vi "Format Event Data.vi"(8 "error in":errorcluster, 9 "event array":T1[](array[typedef]) {"quality" items=["Good"=0, "Good_SubscriptionTransferred"=2949120, "Good_CompletesAsynchronously"=3014656, "Good_Overload"=3080192, "Good_Clamped"=3145728, "Good_LocalOverride"=9830400, "Good_EntryInserted"=10616832, "Good_EntryReplaced"=10682368, "Good_NoData"=10813440, "Good_MoreData"=10878976, "Good_CommunicationEvent"=10944512, "Good_ShutdownEvent"=11010048, "Good_CallAgain"=11075584, "Good_NonCriticalTimeout"=11141120, "Good_ResultsMayBeIncomplete"=12189696, "Good_DataIgnored"=14221312, "Uncertain"=1073741824, "Uncertain_ReferenceOutOfServer"=1080819712, "Uncertain_NoCommunicationLastUsableValue"=1083113472, "Uncertain_LastUsableValue"=1083179008, "Uncertain_SubstituteValue"=1083244544, "Uncertain_InitialValue"=1083310080, "Uncertain_SensorNotAccurate"=1083375616, "Uncertain_EngineeringUnitsExceeded"=1083441152, "Uncertain_SubNormal"=1083506688, "Uncertain_DataSubNormal"=1084489728, "Uncertain_ReferenceNotDeleted"=1086062592, "Uncertain_NotAllNodesAvailable"=1086324736, "Bad"=2147483648, "Bad_UnexpectedError"=2147549184, "Bad_InternalError"=2147614720, "Bad_OutOfMemory"=2147680256, "Bad_ResourceUnavailable"=2147745792, "Bad_CommunicationError"=2147811328, "Bad_EncodingError"=2147876864, "Bad_DecodingError"=2147942400, "Bad_EncodingLimitsExceeded"=2148007936, "Bad_UnknownResponse"=2148073472, "Bad_Timeout"=2148139008, "Bad_ServiceUnsupported"=2148204544, "Bad_Shutdown"=2148270080, "Bad_ServerNotConnected"=2148335616, "Bad_ServerHalted"=2148401152, "Bad_NothingToDo"=2148466688, "Bad_TooManyOperations"=2148532224, "Bad_DataTypeIdUnknown"=2148597760, "Bad_CertificateInvalid"=2148663296, "Bad_SecurityChecksFailed"=2148728832, "Bad_CertificateTimeInvalid"=2148794368, "Bad_CertificateIssuerTimeInvalid"=2148859904, "Bad_CertificateHostNameInvalid"=2148925440, "Bad_CertificateUriInvalid"=2148990976, "Bad_CertificateUseNotAllowed"=2149056512, "Bad_CertificateIssuerUseNotAllowed"=2149122048, "Bad_CertificateUntrusted"=2149187584, "Bad_CertificateRevocationUnknown"=2149253120, "Bad_CertificateIssuerRevocationUnknown"=2149318656, "Bad_CertificateRevoked"=2149384192, "Bad_CertificateIssuerRevoked"=2149449728, "Bad_UserAccessDenied"=2149515264, "Bad_IdentityTokenInvalid"=2149580800, "Bad_IdentityTokenRejected"=2149646336, "Bad_SecureChannelIdInvalid"=2149711872, "Bad_InvalidTimestamp"=2149777408, "Bad_NonceInvalid"=2149842944, "Bad_SessionIdInvalid"=2149908480, "Bad_SessionClosed"=2149974016, "Bad_SessionNotActivated"=2150039552, "Bad_SubscriptionIdInvalid"=2150105088, "Bad_RequestHeaderInvalid"=2150236160, "Bad_TimestampsToReturnInvalid"=2150301696, "Bad_RequestCancelledByClient"=2150367232, "Bad_NoCommunication"=2150694912, "Bad_WaitingForInitialData"=2150760448, "Bad_NodeIdInvalid"=2150825984, "Bad_NodeIdUnknown"=2150891520, "Bad_AttributeIdInvalid"=2150957056, "Bad_IndexRangeInvalid"=2151022592, "Bad_IndexRangeNoData"=2151088128, "Bad_DataEncodingInvalid"=2151153664, "Bad_DataEncodingUnsupported"=2151219200, "Bad_NotReadable"=2151284736, "Bad_NotWritable"=2151350272, "Bad_OutOfRange"=2151415808, "Bad_NotSupported"=2151481344, "Bad_NotFound"=2151546880, "Bad_ObjectDeleted"=2151612416, "Bad_NotImplemented"=2151677952, "Bad_MonitoringModeInvalid"=2151743488, "Bad_MonitoredItemIdInvalid"=2151809024, "Bad_MonitoredItemFilterInvalid"=2151874560, "Bad_MonitoredItemFilterUnsupported"=2151940096, "Bad_FilterNotAllowed"=2152005632, "Bad_StructureMissing"=2152071168, "Bad_EventFilterInvalid"=2152136704, "Bad_ContentFilterInvalid"=2152202240, "Bad_FilterOperandInvalid"=2152267776, "Bad_ContinuationPointInvalid"=2152333312, "Bad_NoContinuationPoints"=2152398848, "Bad_ReferenceTypeIdInvalid"=2152464384, "Bad_BrowseDirectionInvalid"=2152529920, "Bad_NodeNotInView"=2152595456, "Bad_ServerUriInvalid"=2152660992, "Bad_ServerNameMissing"=2152726528, "Bad_DiscoveryUrlMissing"=2152792064, "Bad_SempahoreFileMissing"=2152857600, "Bad_RequestTypeInvalid"=2152923136, "Bad_SecurityModeRejected"=2152988672, "Bad_SecurityPolicyRejected"=2153054208, "Bad_TooManySessions"=2153119744, "Bad_UserSignatureInvalid"=2153185280, "Bad_ApplicationSignatureInvalid"=2153250816, "Bad_NoValidCertificates"=2153316352, "Bad_RequestCancelledByRequest"=2153381888, "Bad_ParentNodeIdInvalid"=2153447424, "Bad_ReferenceNotAllowed"=2153512960, "Bad_NodeIdRejected"=2153578496, "Bad_NodeIdExists"=2153644032, "Bad_NodeClassInvalid"=2153709568, "Bad_BrowseNameInvalid"=2153775104, "Bad_BrowseNameDuplicated"=2153840640, "Bad_NodeAttributesInvalid"=2153906176, "Bad_TypeDefinitionInvalid"=2153971712, "Bad_SourceNodeIdInvalid"=2154037248, "Bad_TargetNodeIdInvalid"=2154102784, "Bad_DuplicateReferenceNotAllowed"=2154168320, "Bad_InvalidSelfReference"=2154233856, "Bad_ReferenceLocalOnly"=2154299392, "Bad_NoDeleteRights"=2154364928, "Bad_ServerIndexInvalid"=2154430464, "Bad_ViewIdUnknown"=2154496000, "Bad_TooManyMatches"=2154627072, "Bad_QueryTooComplex"=2154692608, "Bad_NoMatch"=2154758144, "Bad_MaxAgeInvalid"=2154823680, "Bad_HistoryOperationInvalid"=2154889216, "Bad_HistoryOperationUnsupported"=2154954752, "Bad_WriteNotSupported"=2155020288, "Bad_TypeMismatch"=2155085824, "Bad_MethodInvalid"=2155151360, "Bad_ArgumentsMissing"=2155216896, "Bad_TooManySubscriptions"=2155282432, "Bad_TooManyPublishRequests"=2155347968, "Bad_NoSubscription"=2155413504, "Bad_SequenceNumberUnknown"=2155479040, "Bad_MessageNotAvailable"=2155544576, "Bad_InsufficientClientProfile"=2155610112, "Bad_TcpServerTooBusy"=2155675648, "Bad_TcpMessageTypeInvalid"=2155741184, "Bad_TcpSecureChannelUnknown"=2155806720, "Bad_TcpMessageTooLarge"=2155872256, "Bad_TcpNotEnoughResources"=2155937792, "Bad_TcpInternalError"=2156003328, "Bad_TcpEndpointUrlInvalid"=2156068864, "Bad_RequestInterrupted"=2156134400, "Bad_RequestTimeout"=2156199936, "Bad_SecureChannelClosed"=2156265472, "Bad_SecureChannelTokenUnknown"=2156331008, "Bad_SequenceNumberInvalid"=2156396544, "Bad_ConfigurationError"=2156462080, "Bad_NotConnected"=2156527616, "Bad_DeviceFailure"=2156593152, "Bad_SensorFailure"=2156658688, "Bad_OutOfService"=2156724224, "Bad_DeadbandFilterInvalid"=2156789760, "Bad_RefreshInProgress"=2157379584, "Bad_ConditionAlreadyDisabled"=2157445120, "Bad_ConditionDisabled"=2157510656, "Bad_EventIdUnknown"=2157576192, "Bad_NoData"=2157641728, "Bad_DataLost"=2157772800, "Bad_DataUnavailable"=2157838336, "Bad_EntryExists"=2157903872, "Bad_NoEntryExists"=2157969408, "Bad_TimestampNotSupported"=2158034944, "Bad_InvalidArgument"=2158690304, "Bad_ConnectionRejected"=2158755840, "Bad_Disconnect"=2158821376, "Bad_ConnectionClosed"=2158886912, "Bad_InvalidState"=2158952448, "Bad_EndOfStream"=2159017984, "Bad_NoDataAvailable"=2159083520, "Bad_WaitingForResponse"=2159149056, "Bad_OperationAbandoned"=2159214592, "Bad_ExpectedStreamToBlock"=2159280128, "Bad_WouldBlock"=2159345664, "Bad_SyntaxError"=2159411200, "Bad_MaxConnectionsReached"=2159476736, "Bad_RequestTooLarge"=2159542272, "Bad_ResponseTooLarge"=2159607808, "Bad_EventNotAcknowledgeable"=2159738880, "Bad_InvalidTimestampArgument"=2159869952, "Bad_ProtocolVersionUnsupported"=2159935488, "Bad_StateNotActive"=2160001024, "Bad_FilterOperatorInvalid"=2160132096, "Bad_FilterOperatorUnsupported"=2160197632, "Bad_FilterOperandCountMismatch"=2160263168, "Bad_FilterElementInvalid"=2160328704, "Bad_FilterLiteralInvalid"=2160394240, "Bad_IdentityChangeNotSupported"=2160459776, "Bad_NotTypeDefinition"=2160590848, "Bad_ViewTimestampInvalid"=2160656384, "Bad_ViewParameterMismatch"=2160721920, "Bad_ViewVersionInvalid"=2160787456, "Bad_ConditionAlreadyEnabled"=2160852992, "Bad_DialogNotActive"=2160918528, "Bad_DialogResponseInvalid"=2160984064, "Bad_ConditionBranchAlreadyAcked"=2161049600, "Bad_ConditionBranchAlreadyConfirmed"=2161115136, "Bad_ConditionAlreadyShelved"=2161180672, "Bad_ConditionNotShelved"=2161246208, "Bad_ShelvingTimeOutOfRange"=2161311744, "Bad_AggregateListMismatch"=2161377280, "Bad_AggregateNotSupported"=2161442816, "Bad_AggregateInvalidInputs"=2161508352, "Bad_BoundNotFound"=2161573888, "Bad_BoundNotSupported"=2161639424, "Bad_AggregateConfigurationRejected"=2161770496, "Bad_TooManyMonitoredItems"=2161836032]}, 10 "type":enum16{"Insert", "Replace", "Append"}(ring), 11 "Multicolumn Listbox":refnum<vi>) -> (0 "error out":errorcluster, 1 "Alarm Summary Data":string[][](array[string]), 2 "Alarm Summary Headers":string[](array[string]), 3 "dup Multicolumn Listbox":refnum<vi>)   [LabVIEW 2019]
uses:
  Event Description Item.ctl
  <vilib>/OPCUA/controls/Event Fields.ctl
  <vilib>/OPCUA/controls/NodeId.ctl
  <vilib>/OPCUA/controls/Condition Type.ctl
  <vilib>/OPCUA/controls/OPC UA StatusCode.ctl
panel:
  in  "alarm display format":T5[](array[typedef])=[enum."acked state", enum."confrimed state", enum."time", enum."severity", enum."active", enum."source node ID", enum."condition node ID", enum."condition type", enum."comment", enum."event ID"]
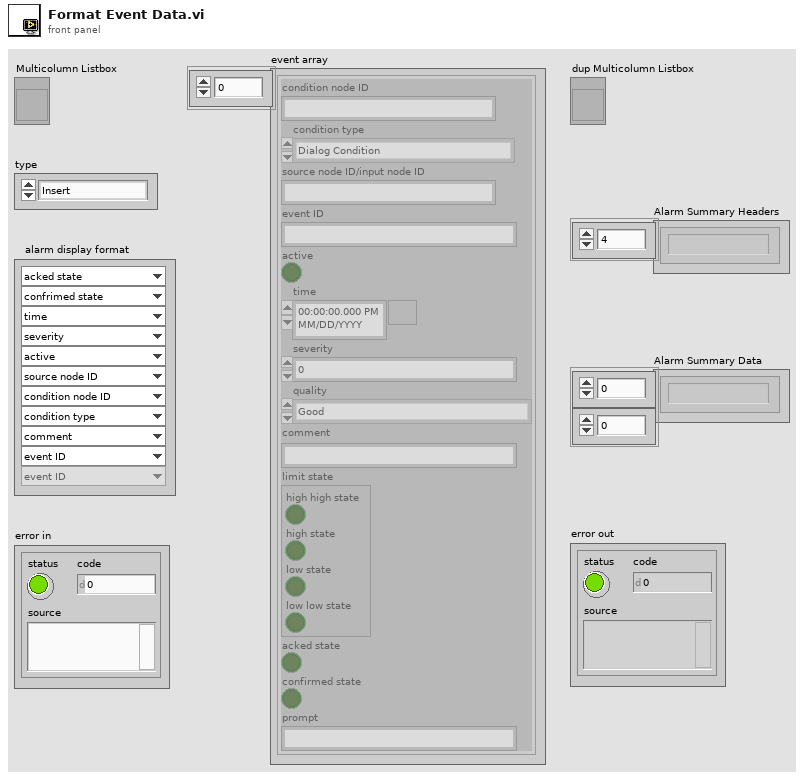
[diagram p1: front panel]
types:
  T1 = typedef "Event Fields.ctl" = cluster{"condition node ID":T2, "condition type":T3, "source node ID/input node ID":T2, "event ID":string, "active":bool, "time":timestamp, "severity":u16, "quality":T4, "comment":string, "limit state":cluster{"high high state":bool, "high state":bool, "low state":bool, "low low state":bool}, "acked state":bool, "confirmed state":bool, "prompt":string}
  T2 = typedef "NodeId.ctl" = string
  T3 = typedef "Condition Type.ctl" = enum16{"Dialog Condition", "Off-Normal Alarm", "Exclusive Level Alarm", "Exclusive Deviation Alarm", "Exclusive Rate of Change Alarm", "Nonexclusive Level Alarm", "Nonexclusive Deviation Alarm", "Nonexclusive Rate of Change Alarm", "Refresh Start Event", "Refresh End Event"}
  T4 = typedef "OPC UA StatusCode.ctl" = u32
  T5 = typedef "Event Description Item.ctl" = enum16{"event ID", "active", "condition type", "condition node ID", "source node ID", "time", "severity", "quality", "comment", "high high state", "high state", "low state", "low low state", "acked state", "confrimed state", "prompt"}
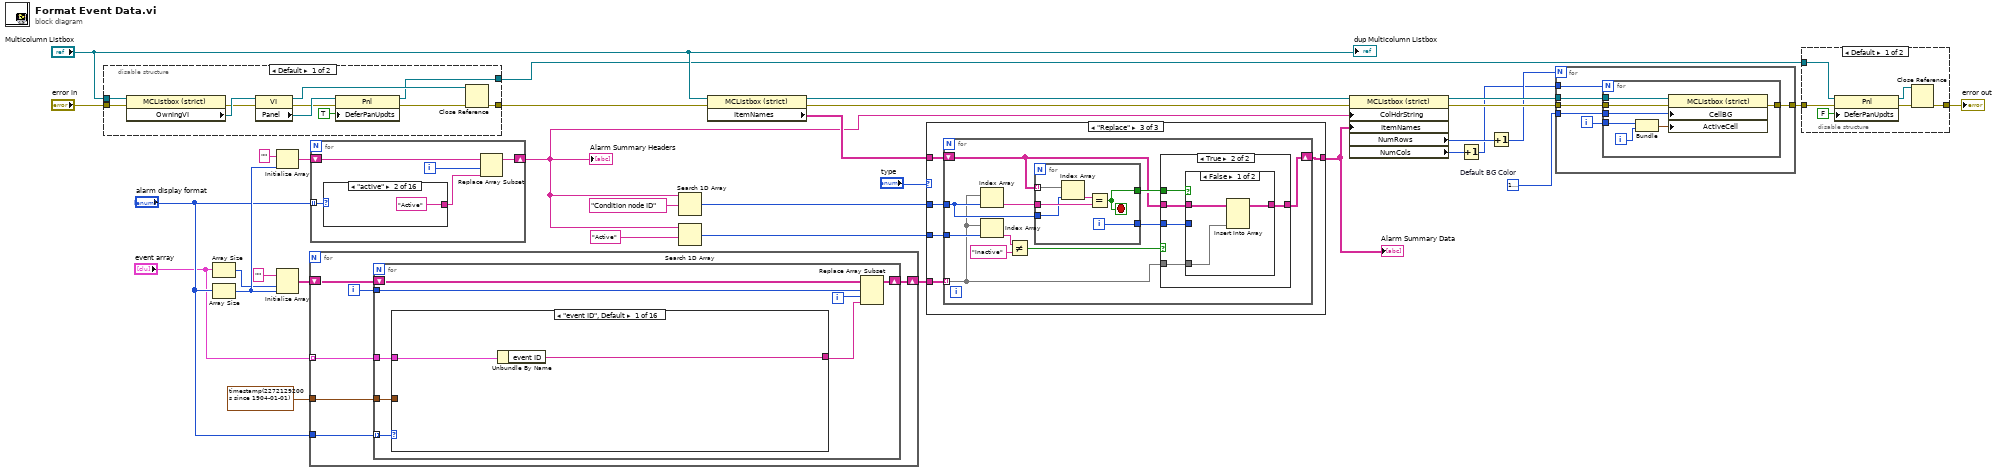
[diagram p0: block diagram]
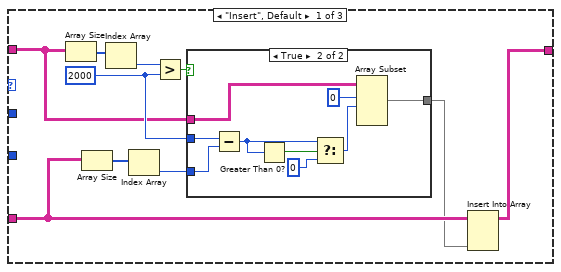
[diagram p4: hidden frame]
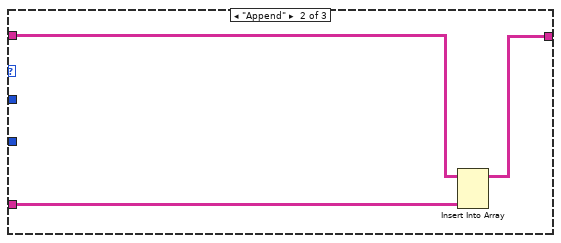
[diagram p6: hidden frame]
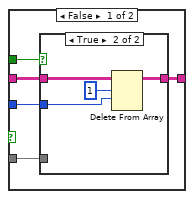
[diagram p7: hidden frame]
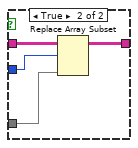
[diagram p9: hidden frame]
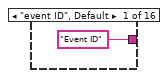
[diagram p10: hidden frame]
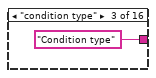
[diagram p11: hidden frame]
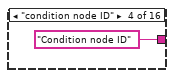
[diagram p12: hidden frame]
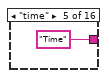
[diagram p13: hidden frame]
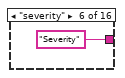
[diagram p14: hidden frame]
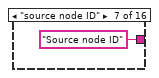
[diagram p15: hidden frame]
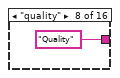
[diagram p16: hidden frame]
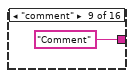
[diagram p17: hidden frame]
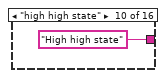
[diagram p18: hidden frame]
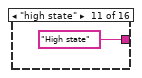
[diagram p19: hidden frame]
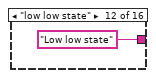
[diagram p20: hidden frame]
diagram:
  w19 = u32 16777226  # Default BG Color
  n1 = disable-structure shown="Default" {
    disable-tunnel: "error in" -> [w37 w45]
    disable-tunnel: "Multicolumn Listbox" -> [w36 _]
    disable-tunnel: [w35 w45] -> w5
    disable-tunnel: [w34 _] -> w2
    frame condition #0 (active) {
      n2 = property class="MCListbox (strict)"(reference=w36, error in=w37) -> (error out=w43:errorcluster, "OwningVI"=w44:refnum<vi>)  [unwired: 1 out]
      n3 = property class="VI"(reference=w44, error in=w43) -> (reference out=w39:refnum<vi>, error out=w41:errorcluster, "Panel"=w42:refnum<vi>)
      n4 = property class="Pnl"(reference=w42, error in=w41, "DeferPanUpdts"=TRUE ("Defer Panel Updates")) -> (reference out=w34:refnum<vi>, error out=w38:errorcluster)
      n5 = Close Reference(reference=w39, error in (no error)=w38) -> (error out=w35:errorcluster)
    }
    frame condition #1 {
    }
  }
  n6 = Array Size(array="event array") -> (size(s)=w28:i32)
  n7 = Array Size(array="alarm display format") -> (size(s)=w32:i32)
  n8 = Initialize Array("" ("element"), w32) -> (w33:string[])
  n9 = Initialize Array("" ("alarm URL"), w28, w32) -> (w30:string[][])
  n10 = for {
    tunnel: "event array" -> [w46] mode=indexing
    tunnel: "alarm display format" -> [w51]
    shift-right: [w49] -> w13
    shift-left: w30 -> [w50]
    tunnel: timestamp(2272129200 s since 1904-01-01) ("ack time") -> [w47]
    i -> [w48]
    n11 = for {
      tunnel: w51 -> [w59] mode=indexing
      tunnel: w46 -> [w52]
      tunnel: w48 -> [w56]
      shift-right: [w57] -> w49
      shift-left: w50 -> [w58]
      tunnel: w47 -> [w53]
      i -> [w55]
      n12 = case shown="\"event ID\", Default" w59 {
        tunnel: w52 -> [w61 w63 w64 w83 w88 w95 w108 w111 w113 w118 w123 w128 w133 w138 w143 w145]
        tunnel: [w60 w62 w65 w82 w87 w94 w106 w109 w112 w114 w119 w124 w129 w134 w139 w144] -> w54
        tunnel: w53 -> [_ _ _ _ w85 _ _ _ _ _ _ _ _ _ _ _]
        frame "event ID", Default {
          n13 = Unbundle By Name(w61) -> ("event ID"=w60:string)
        }
        frame "source node ID" {
          n14 = Unbundle By Name(w63) -> ("source node ID/input node ID"=w62:T2)
        }
        frame "active" {
          n15 = Unbundle By Name(w64) -> ("active"=w66:bool)
          n16 = case shown="True" w66 {
            tunnel: ["Inactive" ("f") w68] -> w65
            tunnel: w64 -> [_ w77]
            frame False {
            }
            frame True {
              n17 = Unbundle By Name(w77) -> ("limit state.high high state"=w76:bool, "limit state.high state"=w75:bool, "limit state.low state"=w74:bool, "limit state.low low state"=w73:bool)
              n18 = Build Array(w76, w75, w74, w73) -> (w72:bool[])
              n19 = Boolean Array To Number(Boolean array=w72) -> (number=w71:u32)
              n20 = case shown="8, 12" w71 {
                tunnel: ["HighHigh" ("f") "High" ("f") "Low" ("f") "LowLow" ("f")] -> w69
                frame 1, 3, Default {
                }
                frame 2 {
                }
                frame 4 {
                }
                frame 8, 12 {
                }
              }
              n21 = Concatenate Strings("Active | " ("f"), w69) -> (w68:string)
            }
          }
        }
        frame "condition node ID" {
          n22 = Unbundle By Name(w83) -> ("condition node ID"=w82:T2)
        }
        frame "time" {
          n23 = Unbundle By Name(w88) -> ("time"=w84:timestamp)
          n24 = Less?(x=w84, y=w85) -> (x < y?=w86:bool)
          n25 = case shown="True" w86 {
            tunnel: w84 -> [w91 _]
            tunnel: [w89 "" ("date/time string")] -> w87
            frame False {
              n26 = Format Date/Time String(time format string (%c)="%m/%d/%Y %H:%M:%S", seconds (now)=w91) -> (date/time string=w89:string)  [unwired: 1 in]
            }
            frame True {
            }
          }
        }
        frame "condition type" {
          n27 = Unbundle By Name(w95) -> ("condition type"=w93:T3)
          n28 = case shown="\"Exclusive Level Alarm\"" w93 {
            tunnel: ["Dialog Condition" ("alarm URL") "Off Normal Alarm" ("alarm URL") "Exclusive Level Alarm" ("alarm URL") "Exclusive Deviation Alarm" ("alarm URL") "Exclusive Rate of Change Alarm" ("alarm URL") "Nonexclusive Level Alarm" ("alarm URL") "Nonexclusive Deviation Alarm" ("alarm URL") "Nonexclusive Rate of Change Alarm" ("alarm URL") "Refresh Start Event" ("alarm URL") "Refresh End Event" ("alarm URL")] -> w94
            frame "Dialog Condition", Default {
            }
            frame "Off-Normal Alarm" {
            }
            frame "Exclusive Level Alarm" {
            }
            frame "Exclusive Deviation Alarm" {
            }
            frame "Exclusive Rate of Change Alarm" {
            }
            frame "Nonexclusive Level Alarm" {
            }
            frame "Nonexclusive Deviation Alarm" {
            }
            frame "Nonexclusive Rate of Change Alarm" {
            }
            frame "Refresh Start Event" {
            }
            frame "Refresh End Event" {
            }
          }
        }
        frame "severity" {
          n29 = Unbundle By Name(w108) -> ("severity"=w107:u16)
          n30 = Number To Decimal String(number=w107) -> (decimal integer string=w106:string)  [unwired: 1 in]
        }
        frame "quality" {
          n31 = Unbundle By Name(w111) -> ("quality"=w110:T4)
          n32 = Number To Decimal String(number=w110) -> (decimal integer string=w109:string)  [unwired: 1 in]
        }
        frame "comment" {
          n33 = Unbundle By Name(w113) -> ("comment"=w112:string)
        }
        frame "high high state" {
          n34 = Unbundle By Name(w118) -> ("limit state.high high state"=w115:bool)
          n35 = Select(t="T" ("alarm URL"), s=w115, f="F") -> (s? t:f=w114:string)
        }
        frame "high state" {
          n36 = Unbundle By Name(w123) -> ("limit state.high state"=w120:bool)
          n37 = Select(t="T" ("alarm URL"), s=w120, f="F") -> (s? t:f=w119:string)
        }
        frame "low low state" {
          n38 = Unbundle By Name(w128) -> ("limit state.low low state"=w125:bool)
          n39 = Select(t="T" ("alarm URL"), s=w125, f="F") -> (s? t:f=w124:string)
        }
        frame "low state" {
          n40 = Unbundle By Name(w133) -> ("limit state.low state"=w130:bool)
          n41 = Select(t="T" ("alarm URL"), s=w130, f="F") -> (s? t:f=w129:string)
        }
        frame "acked state" {
          n42 = Unbundle By Name(w138) -> ("acked state"=w135:bool)
          n43 = Select(t="Yes" ("alarm URL"), s=w135, f="No") -> (s? t:f=w134:string)
        }
        frame "confrimed state" {
          n44 = Unbundle By Name(w143) -> ("confirmed state"=w140:bool)
          n45 = Select(t="Yes" ("alarm URL"), s=w140, f="No") -> (s? t:f=w139:string)
        }
        frame "prompt" {
          n46 = Unbundle By Name(w145) -> ("prompt"=w144:string)
        }
      }
      n47 = Replace Array Subset(array=w58, new element=w54, index (row)=w56, index (col)=w55) -> (w57:string[][])
    }
  }
  n48 = for {
    tunnel: "alarm display format" -> [w150] mode=indexing
    shift-right: [w148] -> w11
    shift-left: w33 -> [w149]
    i -> [w147]
    n49 = case shown="\"active\"" w150 {
      tunnel: ["Event ID" ("element") "Active" ("element") "Condition type" ("element") "Condition node ID" ("element") "Time" ("element") "Severity" ("element") "Source node ID" ("element") "Quality" ("element") "Comment" ("element") "High high state" ("element") "High state" ("element") "Low low state" ("element") "Low state" ("element") "Acked" ("element") "Confirmed" ("element") "Prompt" ("element")] -> w146
      frame "event ID", Default {
      }
      frame "active" {
      }
      frame "condition type" {
      }
      frame "condition node ID" {
      }
      frame "time" {
      }
      frame "severity" {
      }
      frame "source node ID" {
      }
      frame "quality" {
      }
      frame "comment" {
      }
      frame "high high state" {
      }
      frame "high state" {
      }
      frame "low low state" {
      }
      frame "low state" {
      }
      frame "acked state" {
      }
      frame "confrimed state" {
      }
      frame "prompt" {
      }
    }
    n50 = Replace Array Subset(array=w149, new element=w146, index=w147) -> (w148:string[])
  }
  "Alarm Summary Headers" <- w11
  n51 = Search 1D Array(1D array=w11, element="Condition node ID") -> (index of element=w9:i32)  [unwired: 1 in]
  n52 = Search 1D Array(1D array=w11, element="Active") -> (index of element=w8:i32)  [unwired: 1 in]
  n53 = property class="MCListbox (strict)"(reference="Multicolumn Listbox", error in=w5) -> (reference out=w16:refnum<vi>, error out=w17:errorcluster, "ItemNames"=w14:string[][])
  n54 = case shown="\"Replace\"" "type" {
    tunnel: w14 -> [w167 w187 w193]
    tunnel: w13 -> [w173 w188 w194]
    tunnel: [w174 w189 w190] -> w12
    tunnel: w9 -> [_ _ w192]
    tunnel: w8 -> [_ _ w191]
    frame "Insert", Default {
      w169 = 2000 ("y")
      n55 = Array Size(array=w167) -> (size(s)=w176:i32[])
      n56 = Array Size(array=w173) -> (size(s)=w172:i32[])
      n57 = Index Array(array=w176) -> (element=w170:i32)  [unwired: 1 in]
      n58 = Index Array(array=w172) -> (element=w171:i32)  [unwired: 1 in]
      n59 = Greater?(x=w170, y=w169) -> (0:w175:bool)
      n60 = case shown="True" w175 {
        tunnel: w167 -> [w177 w186]
        tunnel: w171 -> [_ w184]
        tunnel: w169 -> [_ w185]
        tunnel: [w177 w178] -> w168
        frame False {
        }
        frame True {
          n61 = Subtract(x=w185, y=w184) -> (x-y=w182:i32)
          n62 = Greater Than 0?(x=w182) -> (x > 0?=w183:bool)
          n63 = Select(t=w182, s=w183, f=0) -> (s? t:f=w179:i32)
          n64 = Array Subset(array=w186, index (row)=0, length (row)=w179) -> (w178:string[][])  [unwired: 2 in]
        }
      }
      n65 = Insert Into Array(array=w173, new element=w168) -> (w174:string[][])  [unwired: 2 in]
    }
    frame "Append" {
      n66 = Insert Into Array(array=w187, new element=w188) -> (w189:string[][])  [unwired: 2 in]
    }
    frame "Replace" {
      n67 = for {
        tunnel: w194 -> [w196] mode=indexing
        tunnel: w192 -> [w197]
        tunnel: w191 -> [w198]
        shift-right: [w195] -> w190
        shift-left: w193 -> [w199]
        n68 = Index Array(array=w196, index=w197) -> (element=w205:string)
        n69 = Index Array(array=w196, index=w198) -> (element=w203:string)
        n70 = Not Equal?(x=w203, y="Inactive" ("f")) -> (x != y?=w201:bool)
        n71 = for {
          tunnel: [w233] -> w202
          tunnel: [w232] -> w200
          tunnel: w199 -> [w231] mode=indexing
          tunnel: w205 -> [w229]
          tunnel: w197 -> [w228]
          i -> [w232]
          stop <- w233 stop-if-true
          n72 = Index Array(array=w231, index=w228) -> (element=w230:string)
          n73 = Equal?(x=w230, y=w229) -> (x = y?=w233:bool)
        }
        n74 = case shown="True" w201 {
          tunnel: w202 -> [w210 w220]
          tunnel: w200 -> [w206 w219]
          tunnel: w199 -> [w208 w218]
          tunnel: w196 -> [w209 w217]
          tunnel: [w207 w216] -> w195
          frame False {
            n75 = case shown="True" w210 {
              tunnel: w209 -> [_ _]
              tunnel: w208 -> [w211 w215]
              tunnel: [w211 w213] -> w207
              tunnel: w206 -> [_ w212]
              frame False {
              }
              frame True {
                n76 = Delete From Array(array=w215, length=1, index (row)=w212) -> (array with subset deleted=w213:string[][])  [unwired: 1 in, 1 out]
              }
            }
          }
          frame True {
            n77 = case shown="False" w220 {
              tunnel: w219 -> [_ w226]
              tunnel: w218 -> [w223 w227]
              tunnel: w217 -> [w222 w225]
              tunnel: [w221 w224] -> w216
              frame False {
                n78 = Insert Into Array(array=w223, new element=w222) -> (w221:string[][])  [unwired: 2 in]
              }
              frame True {
                n79 = Replace Array Subset(array=w227, new element=w225, index (row)=w226) -> (w224:string[][])  [unwired: 1 in]
              }
            }
          }
        }
      }
    }
  }
  "Alarm Summary Data" <- w12
  n80 = property class="MCListbox (strict)"(reference=w16, error in=w17, "ColHdrString"=w11, "ItemNames"=w12) -> (reference out=w24:refnum<vi>, error out=w23:errorcluster, "NumRows"=w25:u32, "NumCols"=w26:u32)
  n81 = Increment(x=w26) -> (x+1=w20:u32)
  n82 = Increment(x=w25) -> (x+1=w21:u32)
  n83 = for {
    N: w21 -> [_]
    tunnel: [w238] -> w4
    tunnel: w20 -> [w237]
    tunnel: w24 -> [w236]
    tunnel: w19 -> [w235]
    tunnel: w23 -> [w234]
    i -> [w239]
    n84 = for {
      N: w237 -> [_]
      tunnel: w239 -> [w246]
      tunnel: [w245] -> w238
      tunnel: w236 -> [w243]
      tunnel: w235 -> [w242]
      tunnel: w234 -> [w241]
      i -> [w244]
      n85 = Bundle(w246, w244) -> (w240:cluster{i32, i32})  [unwired: 1 in]
      n86 = property class="MCListbox (strict)"(reference=w243, error in=w241, "CellBG"=w242, "ActiveCell"=w240) -> (error out=w245:errorcluster)  [unwired: 1 out]
    }
  }
  n87 = disable-structure shown="Default" {
    disable-tunnel: w4 -> [w249 w253]
    disable-tunnel: [w248 w253] -> w3
    disable-tunnel: w2 -> [w247 _]
    frame condition #0 (active) {
      n88 = property class="Pnl"(reference=w247, error in=w249, "DeferPanUpdts"=FALSE ("Defer Panel Updates")) -> (reference out=w250:refnum<vi>, error out=w251:errorcluster)
      n89 = Close Reference(reference=w250, error in (no error)=w251) -> (error out=w248:errorcluster)
    }
    frame condition #1 {
    }
  }
  "error out" <- w3
  "dup Multicolumn Listbox" <- "Multicolumn Listbox"
